vi "Find_Pos(Index)_Particle_in_(X,Y)-2.vi"(1 "[X,Y] (n Frame)":dbl[](array[numeric]), 2 "Y1":dbl, 3 "X1":dbl) -> (0 "Index in (n) Frame":i32)   [LabVIEW 2013]
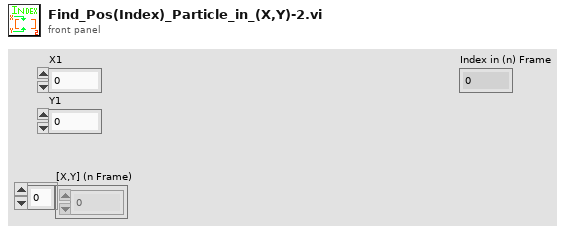
[diagram p1: front panel]
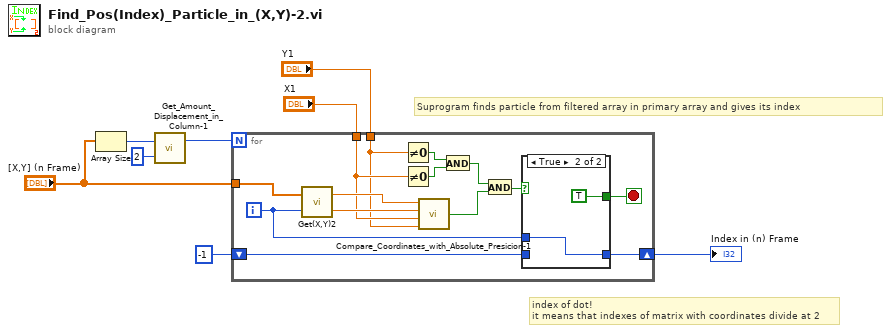
[diagram p0: block diagram]
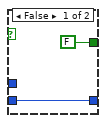
[diagram p2: hidden frame]
diagram:
  # "index of dot! \nit means that indexes of matrix with coordinates divide at 2"
  # "Suprogram finds particle from filtered array in primary array and gives its index"
  n1 = Array Size(array="[X,Y] (n Frame)") -> (size(s)=w3:i32)
  n2 = call "Get_Amount_Displacement_in_Column-1.vi"("multiplier"=2 ("y"), "# Rows"=w3) -> ("Displ amount"=w1:i32)  [unwired: 1 out]
  n3 = for {
    N: w1 -> [_]
    tunnel: "[X,Y] (n Frame)" -> [w16]
    shift-right: [w17] -> w4
    shift-left: -1 -> [w18]
    tunnel: "X1" -> [w11]
    tunnel: "Y1" -> [w10]
    i -> [w15]
    stop <- w14 stop-if-true
    n4 = call "Get(X,Y)2.vi"("[IN] index of (X,Y)"=w15, "[IN] Array coordi\nnates (X,Y) in Frame"=w16) -> ("[OUT] Y"=w12:dbl, "[OUT] X"=w13:dbl)
    n5 = Not Equal To 0?(x=w10) -> (x != 0?=w22:bool)
    n6 = Not Equal To 0?(x=w11) -> (x != 0?=w21:bool)
    n7 = call "Compare_Coordinates_with_Absolute_Presicion-1.vi"("X 1"=w13, "Y 1"=w12, "X 2"=w11, "Y 2"=w10) -> ("[OUT] Same coordinates?"=w9:bool)  [unwired: 1 in]
    n8 = And(x=w22, y=w21) -> (x .and. y?=w20:bool)
    n9 = And(x=w20, y=w9) -> (x .and. y?=w19:bool)
    n10 = case shown="True" w19 {
      tunnel: w18 -> [w24 _]
      tunnel: w15 -> [_ w26]
      tunnel: [w24 w26] -> w17
      tunnel: [FALSE TRUE] -> w14
      frame False {
      }
      frame True {
      }
    }
  }
  "Index in (n) Frame" <- w4
